vi "Begin.vi"(8 "error in":errorcluster) -> (0 "error out":errorcluster)   [LabVIEW 2019]
doc: "Called before other user functions, this VI is expected to open initial I/O refnums, load in file data, and do all program initialization. Notice that the <B>error out</B> terminal is simply used for data flow. Wiring it to other structures or subVIs ensures that this VI runs first."
uses:
  <vilib>/Rock Robotics/WPI/DriverStation/WPI_DriverStationRobotMode2.ctl
  <vilib>/Rock Robotics/WPI/Joystick/WPI_JoystickDeviceEnum.ctl
  <vilib>/Rock Robotics/SystemInterfaces/i2clib/i2c_bus.ctl
  <vilib>/Rock Robotics/WPI/Solenoid/WPI_SolenoidChannel.ctl
  <vilib>/Rock Robotics/WPI/ThirdParty/Phoenix-LabVIEW/Motor Controller/Controls/CTRE_Phoenix_MotorControl_LimitSwitchSource_Local.ctl
  <vilib>/Rock Robotics/WPI/ThirdParty/Phoenix-LabVIEW/Motor Controller/Controls/CTRE_Phoenix_MotorControl_LimitSwitchNormal.ctl
  <vilib>/Rock Robotics/SystemInterfaces/DIO/FPGA_DIOChannel.ctl
  Robot Global Data.vi
  <vilib>/Rock Robotics/Network Tables/NT Write String Array.vi
  <vilib>/Rock Robotics/WPI/Ultrasonic/WPI_SonarSRF04DigitalOpen.vi
  <vilib>/Rock Robotics/WPI/Ultrasonic/WPI_SonarSRF04DigitalRefNum Registry Set.vi
  <vilib>/Rock Robotics/WPI/Utilities/WPI_GetSetVariantRefNum.vi
  <vilib>/Rock Robotics/WPI/Switch/WPI_SwitchOpenLimit.vi
  <vilib>/Rock Robotics/WPI/Solenoid/WPI_SolenoidOpenDouble.vi
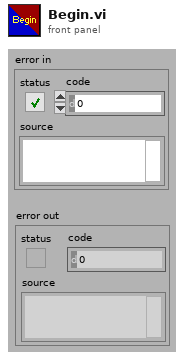
[diagram p1: front panel]
types:
  T1 = typedef "FPGA_DIOChannel.ctl" = enum8{"DIO 0", "DIO 1", "DIO 2", "DIO 3", "DIO 4", "DIO 5", "DIO 6", "DIO 7", "DIO 8", "DIO 9", "DIO MXP 0", "DIO MXP 1", "DIO MXP 2", "DIO MXP 3", "DIO MXP 4", "DIO MXP 5", "DIO MXP 6", "DIO MXP 7", "DIO MXP 8", "DIO MXP 9", "DIO MXP 10", "DIO MXP 11", "DIO MXP 12", "DIO MXP 13", "DIO MXP 14", "DIO MXP 15", "SPI Port CS1", "SPI Port CS2", "SPI Port CS3", "SPI Port MISO", "SPI Port MOSI", "Invalid"}
  T2 = typedef "WPI_SolenoidChannel.ctl" = enum8{"Solenoid 0", "Solenoid 1", "Solenoid 2", "Solenoid 3", "Solenoid 4", "Solenoid 5", "Solenoid 6", "Solenoid 7", "Invalid"}
  T3 = typedef "CTRE_Phoenix_MotorControl_LimitSwitchNormal.ctl" = enum16{"Normally Open", "Normally Closed", "Disabled"}
  T4 = typedef "CTRE_Phoenix_MotorControl_LimitSwitchSource_Local.ctl" = enum16{"Feedback Connector", "Remote Talon SRX", "Remote CANifier", "Deactivated"}
  T5 = typedef "WPI_JoystickDeviceEnum.ctl" = enum16{"USB 0", "USB 1", "USB 2", "USB 3", "USB 4", "USB 5"}
  T6 = typedef "i2c_bus.ctl" = enum16{"I2C On-Board", "I2C MXP", "Invalid"}
  T7 = typedef "WPI_DriverStationRobotMode2.ctl" = enum16{"Autonomous Disabled", "Autonomous Enabled", "Teleop Disabled", "Teleop Enabled", "Disconnected", "Finish", "Test Disabled", "Test Enabled", "Emergency Stopped"}
  T8 = typedef "WPI_CompressorDevRef.ctl" = cluster{"DevStatus":errorcluster, "Pneumatics Control Module":u8}
  T9 = typedef "WPI_SwitchDevRef.ctl" = cluster{"DevStatus":errorcluster, "DIO Channel":T1, "CntIndex":T10, "Normally Closed":bool}
  T10 = typedef "FPGA_CounterCtrSystemIndex.ctl" = enum8{"Ctr 0", "Ctr 1", "Ctr 2", "Ctr 3", "Ctr 4", "Ctr 5", "Ctr 6", "Ctr 7", "Invalid"}
  T11 = typedef "WPI_UltrasonicDeviceRef.ctl" = cluster{"DevStatus":errorcluster, "Ping Channel":T1, "Echo Channel":T1, "CntIndex":T10}
  T12 = typedef "Color Sensor V3 DevRef.ctl" = cluster{"I2CDevRef":T13}
  T13 = typedef "WPI_I2CDevRef.ctl" = cluster{"DevStatus":errorcluster, "Device Address":u8, "Handle":i32, "I2C Bus":T6}
  T14 = typedef "WPI_SolenoidDevRef.ctl" = cluster{"DevStatus":errorcluster, "Pneumatics Control Module":u8, "Forward Solenoid Channel":T2, "Reverse Solenoid Channel":T2}
  T15 = typedef "WPI_MotorControlDeviceRef.ctl" = cluster{"DeviceStatus":errorcluster, "Type":T16, "PWM":cluster{"PWM Channel":T17, "DeadBand":T18}, "CAN":cluster{"Device Number":u8, "SetOutput VI Ref":variant, "GetOutput VI Ref":variant, "Enable VI Ref":variant, "Disable VI Ref":variant, "Data":variant}, "Invert":bool, "DIO PWM":cluster{"PWM \"Enable\" Channel":T17, "DIOChannel":T1, "PWM Rate":dbl}}
  T16 = typedef "WPI_MotorControlType.ctl" = enum16{"PWM", "CAN", "DIO PWM"}
  T17 = typedef "FPGA_DIOPWMChannel.ctl" = enum8{"PWM 0", "PWM 1", "PWM 2", "PWM 3", "PWM 4", "PWM 5", "PWM 6", "PWM 7", "PWM 8", "PWM 9", "PWM MXP 0", "PWM MXP 1", "PWM MXP 2", "PWM MXP 3", "PWM MXP 4", "PWM MXP 5", "PWM MXP 6", "PWM MXP 7", "PWM MXP 8", "PWM MXP 9", "Invalid"}
  T18 = typedef "WPI_PWMDeadband.ctl" = cluster{"Name":string, "maxPositivePwm":i32, "minPositivePwm":i32, "centerPwm":i32, "maxNegativePwm":i32, "minNegativePwm":i32, "angularRange":u16}
  T19 = typedef "WPI_JoystickDevRef.ctl" = cluster{"Device":T5}
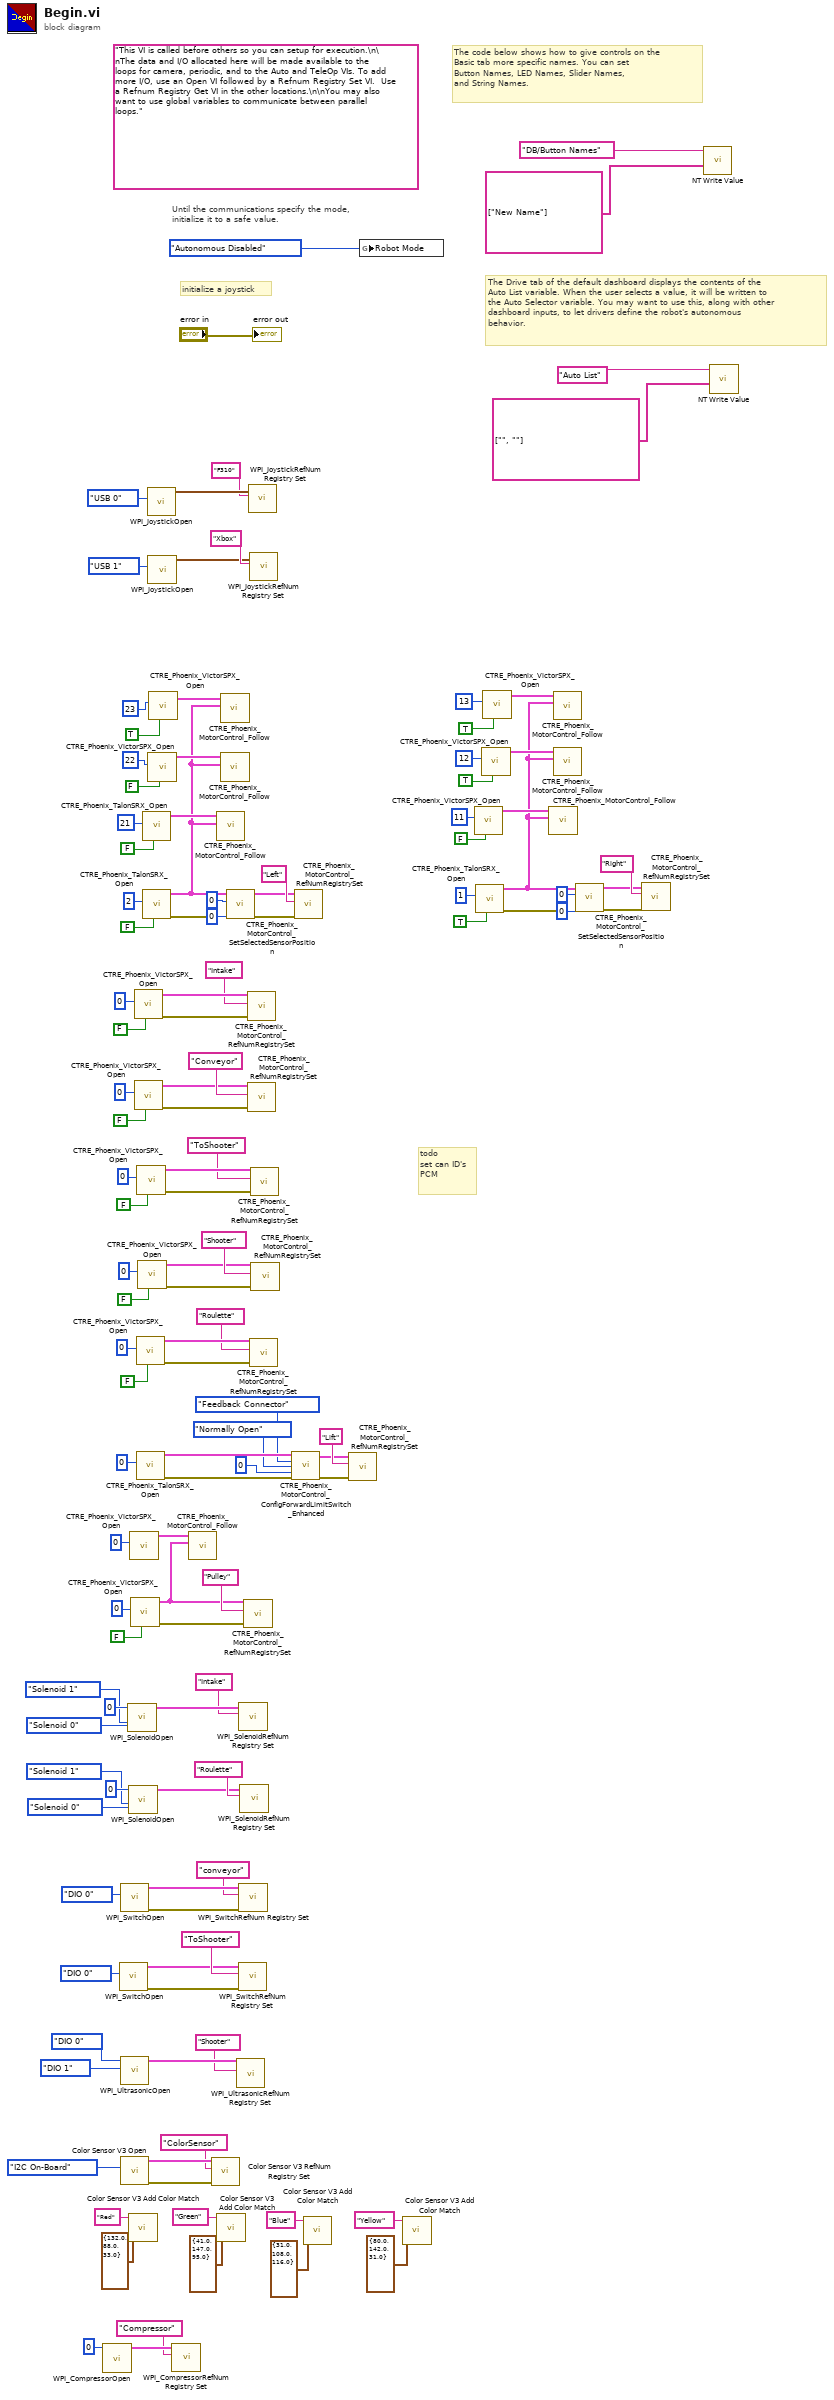
[diagram p0: block diagram]
diagram:
  (unwired) "This VI is called before others so you can setup for execution.\n\nThe data and I/O allocated here will be made available to the loops for camera, periodic, and to the Auto and TeleOp VIs. To add more I/O, use an Open VI followed by a Refnum Registry Set VI.  Use a Refnum Registry Get VI in the other locations.\n\nYou may also want to use global variables to communicate between parallel loops."
  # "todo\nset can ID's\nPCM"
  # "The Drive tab of the default dashboard displays the contents of the\nAuto List variable. When the user selects a value, it will be written to\nthe Auto Selector variable. You may want to use this, along with other\ndashboard inputs, to let drivers define the robot's autonomous\nbehavior."
  # "The code below shows how to give controls on the\nBasic tab more specific names. You can set\nButton Names, LED Names, Slider Names,\nand String Names."
  # "initialize a joystick"
  # "Until the communications specify the mode,\ninitialize it to a safe value."
  n1 = call <vilib>:"WPI_CompressorOpen.vi"("Pneumatics Control Module (0)"=u8 0) -> ("CompressorDevRef"=w11:T8)  [unwired: 13 in, 1 out]
  n2 = call-poly <vilib>:"WPI_SwitchOpen.vi"("DIO Channel"=FPGA_DIOChannel."DIO 0") -> ("error out"=w1:errorcluster, "SwitchDevRef"=w2:T9)  [unwired: 9 in]
  n3 = call-poly <vilib>:"WPI_SwitchOpen.vi"("DIO Channel"=FPGA_DIOChannel."DIO 0") -> ("error out"=w27:errorcluster, "SwitchDevRef"=w26:T9)  [unwired: 9 in]
  n4 = call-poly <vilib>:"WPI_UltrasonicOpen.vi"("Echo DIO Channel"=FPGA_DIOChannel."DIO 1", "Ping DIO Channel"=FPGA_DIOChannel."DIO 0") -> ("SonarSRF04DevRef"=w14:T11)  [unwired: 8 in, 1 out]
  n5 = call <vilib>:"Color Sensor V3 Open.vi"("I2C Bus"=i2c_bus."I2C On-Board") -> ("error out"=w84:errorcluster, "ColorSensorDevRef"=w83:T12)  [unwired: 9 in]
  n6 = call-poly <vilib>:"WPI_SolenoidOpen.vi"("Reverse Solenoid Channel"=WPI_SolenoidChannel."Solenoid 1", "Forward Solenoid Channel"=WPI_SolenoidChannel."Solenoid 0", "Pneumatics Control Module (0)"=u8 0) -> ("SolenoidDevRef"=w39:T14)  [unwired: 7 in, 1 out]
  n7 = call-poly <vilib>:"WPI_SolenoidOpen.vi"("Reverse Solenoid Channel"=WPI_SolenoidChannel."Solenoid 1", "Forward Solenoid Channel"=WPI_SolenoidChannel."Solenoid 0", "Pneumatics Control Module (0)"=u8 0) -> ("SolenoidDevRef"=w36:T14)  [unwired: 7 in, 1 out]
  n8 = call <vilib>:"Color Sensor V3 Add Color Match.vi"("Color"=cluster{"R":dbl, "G":dbl, "B":dbl} {"R"=132.0, "G"=88.0, "B"=33.0}, "Name"="Red") -> ()  [unwired: 10 in]
  n9 = call <vilib>:"CTRE_Phoenix_VictorSPX_Open.vi"("Device Number"=u8 0) -> ("CAN Talon SRX Ref"=w43:T15)  [unwired: 9 in, 1 out]
  n10 = call <vilib>:"CTRE_Phoenix_VictorSPX_Open.vi"("Invert"=FALSE, "Device Number"=u8 0) -> ("error out"=w45:errorcluster, "CAN Talon SRX Ref"=w42:T15)  [unwired: 8 in]
  n11 = call <vilib>:"CTRE_Phoenix_VictorSPX_Open.vi"("Invert"=FALSE, "Device Number"=u8 0) -> ("error out"=w92:errorcluster, "CAN Talon SRX Ref"=w91:T15)  [unwired: 8 in]
  n12 = call <vilib>:"CTRE_Phoenix_VictorSPX_Open.vi"("Invert"=FALSE, "Device Number"=u8 0) -> ("error out"=w60:errorcluster, "CAN Talon SRX Ref"=w61:T15)  [unwired: 8 in]
  n13 = call <vilib>:"CTRE_Phoenix_VictorSPX_Open.vi"("Invert"=FALSE, "Device Number"=u8 0) -> ("error out"=w30:errorcluster, "CAN Talon SRX Ref"=w29:T15)  [unwired: 8 in]
  n14 = call <vilib>:"CTRE_Phoenix_TalonSRX_Open.vi"("Device Number"=u8 0) -> ("error out"=w22:errorcluster, "CAN Talon SRX Ref"=w19:T15)  [unwired: 9 in]
  n15 = call <vilib>:"CTRE_Phoenix_VictorSPX_Open.vi"("Invert"=FALSE, "Device Number"=u8 0) -> ("error out"=w55:errorcluster, "CAN Talon SRX Ref"=w54:T15)  [unwired: 8 in]
  n16 = call <vilib>:"CTRE_Phoenix_VictorSPX_Open.vi"("Invert"=FALSE, "Device Number"=u8 0) -> ("error out"=w50:errorcluster, "CAN Talon SRX Ref"=w51:T15)  [unwired: 8 in]
  n17 = call <vilib>:"CTRE_Phoenix_TalonSRX_Open.vi"("Invert"=FALSE, "Device Number"=u8 21) -> ("CAN Talon SRX Ref"=w117:T15)  [unwired: 8 in, 1 out]
  n18 = call <vilib>:"CTRE_Phoenix_TalonSRX_Open.vi"("Invert"=FALSE, "Device Number"=u8 2) -> ("error out"=w65:errorcluster, "CAN Talon SRX Ref"=w68:T15)  [unwired: 8 in]
  n19 = call <vilib>:"WPI_JoystickOpen.vi"("JoystickDevice"=WPI_JoystickDeviceEnum."USB 0") -> ("JoystickDevRef"=w96:T19)  [unwired: 10 in]
  n20 = call <vilib>:"WPI_JoystickOpen.vi"("JoystickDevice"=WPI_JoystickDeviceEnum."USB 1") -> ("JoystickDevRef"=w72:T19)  [unwired: 10 in]
  n21 = call <vilib>:"CTRE_Phoenix_VictorSPX_Open.vi"("Invert"=FALSE, "Device Number"=u8 22) -> ("CAN Talon SRX Ref"=w112:T15)  [unwired: 8 in, 1 out]
  n22 = call <vilib>:"CTRE_Phoenix_VictorSPX_Open.vi"("Invert"=TRUE, "Device Number"=u8 23) -> ("CAN Talon SRX Ref"=w111:T15)  [unwired: 8 in, 1 out]
  n23 = call <vilib>:"WPI_CompressorRefNum Registry Set.vi"("refnum name"="Compressor", "CompressorDevRef"=w11) -> ()  [unwired: 8 in, 2 out]
  n24 = call <vilib>:"CTRE_Phoenix_MotorControl_Follow.vi"("Master Controller to Follow"=w42, "PhoenixMotorControlDevRef"=w43) -> ()  [unwired: 8 in, 2 out]
  n25 = call <vilib>:"Color Sensor V3 RefNum Registry Set.vi"("error in (no error)"=w84, "refnum name"="ColorSensor", "ColorSensorDevRef"=w83) -> ()  [unwired: 7 in, 2 out]
  n26 = call <vilib>:"CTRE_Phoenix_MotorControl_Follow.vi"("Master Controller to Follow"=w68, "PhoenixMotorControlDevRef"=w117) -> ()  [unwired: 8 in, 2 out]
  n27 = call <vilib>:"Color Sensor V3 Add Color Match.vi"("Color"=cluster{"R":dbl, "G":dbl, "B":dbl} {"R"=41.0, "G"=147.0, "B"=95.0}, "Name"="Green") -> ()  [unwired: 10 in]
  n28 = call <vilib>:"CTRE_Phoenix_MotorControl_Follow.vi"("Master Controller to Follow"=w68, "PhoenixMotorControlDevRef"=w111) -> ()  [unwired: 8 in, 2 out]
  n29 = call <vilib>:"CTRE_Phoenix_MotorControl_Follow.vi"("Master Controller to Follow"=w68, "PhoenixMotorControlDevRef"=w112) -> ()  [unwired: 8 in, 2 out]
  n30 = call <vilib>:"CTRE_Phoenix_MotorControl_SetSelectedSensorPosition.vi"("error in (no error)"=w65, "pidLoopIdx"=u32 0, "New Sensor Position"=0, "PhoenixMotorControlDevRef"=w68) -> ("error out"=w66:errorcluster, "PhoenixMotorControlDevRef"=w67:T15)  [unwired: 6 in]
  n31 = call-poly <vilib>:"WPI_UltrasonicRefNum Registry Set.vi"("refnum name"="Shooter", "SonarSRF04DevRef"=w14) -> ()  [unwired: 8 in, 2 out]
  n32 = call <vilib>:"WPI_SwitchRefNum Registry Set.vi"("error in (no error)"=w1, "refnum name"="ToShooter", "SwitchDevRef"=w2) -> ()  [unwired: 7 in, 2 out]
  n33 = call <vilib>:"WPI_SolenoidRefNum Registry Set.vi"("refnum name"="Intake", "SolenoidDevRef"=w39) -> ()  [unwired: 8 in, 2 out]
  n34 = call <vilib>:"WPI_SwitchRefNum Registry Set.vi"("error in (no error)"=w27, "refnum name"="conveyor", "SwitchDevRef"=w26) -> ()  [unwired: 7 in, 2 out]
  n35 = call <vilib>:"WPI_SolenoidRefNum Registry Set.vi"("refnum name"="Roulette", "SolenoidDevRef"=w36) -> ()  [unwired: 8 in, 2 out]
  n36 = call <vilib>:"CTRE_Phoenix_MotorControl_RefNumRegistrySet.vi"("error in (no error)"=w45, "refnum name"="Pulley", "PhoenixMotorControlDevRef"=w42) -> ()  [unwired: 7 in, 2 out]
  n37 = call <vilib>:"CTRE_Phoenix_MotorControl_RefNumRegistrySet.vi"("error in (no error)"=w92, "refnum name"="Intake", "PhoenixMotorControlDevRef"=w91) -> ()  [unwired: 7 in, 2 out]
  n38 = call <vilib>:"CTRE_Phoenix_MotorControl_RefNumRegistrySet.vi"("error in (no error)"=w60, "refnum name"="Conveyor", "PhoenixMotorControlDevRef"=w61) -> ()  [unwired: 7 in, 2 out]
  n39 = call <vilib>:"WPI_JoystickRefNum Registry Set.vi"("refnum name"="F310", "JoystickDevRef"=w96) -> ()  [unwired: 8 in, 2 out]
  n40 = call <vilib>:"WPI_JoystickRefNum Registry Set.vi"("refnum name"="Xbox", "JoystickDevRef"=w72) -> ()  [unwired: 8 in, 2 out]
  n41 = call <vilib>:"CTRE_Phoenix_MotorControl_RefNumRegistrySet.vi"("error in (no error)"=w30, "refnum name"="Roulette", "PhoenixMotorControlDevRef"=w29) -> ()  [unwired: 7 in, 2 out]
  n42 = call <vilib>:"CTRE_Phoenix_MotorControl_RefNumRegistrySet.vi"("error in (no error)"=w55, "refnum name"="ToShooter", "PhoenixMotorControlDevRef"=w54) -> ()  [unwired: 7 in, 2 out]
  n43 = call <vilib>:"CTRE_Phoenix_MotorControl_RefNumRegistrySet.vi"("error in (no error)"=w50, "refnum name"="Shooter", "PhoenixMotorControlDevRef"=w51) -> ()  [unwired: 7 in, 2 out]
  n44 = call <vilib>:"CTRE_Phoenix_MotorControl_ConfigForwardLimitSwitch_Enhanced.vi"("PhoenixMotorControlDevRef"=w19, "Limit Switch Source"=CTRE_Phoenix_MotorControl_LimitSwitchSource_Local."Feedback Connector", "NormallyOpenOrClosed"=CTRE_Phoenix_MotorControl_LimitSwitchNormal."Normally Open", "deviceID"=0, "error in (no error)"=w22) -> ("PhoenixMotorControlDevRef"=w20:T15, "error out"=w21:errorcluster)  [unwired: 9 in]
  n45 = call <vilib>:"CTRE_Phoenix_MotorControl_RefNumRegistrySet.vi"("error in (no error)"=w66, "refnum name"="Left", "PhoenixMotorControlDevRef"=w67) -> ()  [unwired: 7 in, 2 out]
  n46 = call <vilib>:"Color Sensor V3 Add Color Match.vi"("Color"=cluster{"R":dbl, "G":dbl, "B":dbl} {"R"=31.0, "G"=108.0, "B"=116.0}, "Name"="Blue") -> ()  [unwired: 10 in]
  n47 = call <vilib>:"CTRE_Phoenix_MotorControl_RefNumRegistrySet.vi"("error in (no error)"=w21, "refnum name"="Lift", "PhoenixMotorControlDevRef"=w20) -> ()  [unwired: 7 in, 2 out]
  n48 = global write "Robot Global Data.vi" "Robot Mode"(WPI_DriverStationRobotMode2."Autonomous Disabled" ("Robot Mode")) -> ()
  n49 = call <vilib>:"Color Sensor V3 Add Color Match.vi"("Color"=cluster{"R":dbl, "G":dbl, "B":dbl} {"R"=80.0, "G"=142.0, "B"=31.0}, "Name"="Yellow") -> ()  [unwired: 10 in]
  n50 = call <vilib>:"CTRE_Phoenix_VictorSPX_Open.vi"("Invert"=FALSE, "Device Number"=u8 11) -> ("CAN Talon SRX Ref"=w100:T15)  [unwired: 8 in, 1 out]
  n51 = call <vilib>:"CTRE_Phoenix_TalonSRX_Open.vi"("Invert"=TRUE, "Device Number"=u8 1) -> ("error out"=w64:errorcluster, "CAN Talon SRX Ref"=w89:T15)  [unwired: 8 in]
  n52 = call <vilib>:"CTRE_Phoenix_VictorSPX_Open.vi"("Invert"=TRUE, "Device Number"=u8 12) -> ("CAN Talon SRX Ref"=w109:T15)  [unwired: 8 in, 1 out]
  n53 = call <vilib>:"CTRE_Phoenix_VictorSPX_Open.vi"("Invert"=TRUE, "Device Number"=u8 13) -> ("CAN Talon SRX Ref"=w110:T15)  [unwired: 8 in, 1 out]
  n54 = call <vilib>:"CTRE_Phoenix_MotorControl_Follow.vi"("Master Controller to Follow"=w89, "PhoenixMotorControlDevRef"=w100) -> ()  [unwired: 8 in, 2 out]
  n55 = call <vilib>:"CTRE_Phoenix_MotorControl_Follow.vi"("Master Controller to Follow"=w89, "PhoenixMotorControlDevRef"=w110) -> ()  [unwired: 8 in, 2 out]
  n56 = call <vilib>:"CTRE_Phoenix_MotorControl_Follow.vi"("Master Controller to Follow"=w89, "PhoenixMotorControlDevRef"=w109) -> ()  [unwired: 8 in, 2 out]
  n57 = call <vilib>:"CTRE_Phoenix_MotorControl_SetSelectedSensorPosition.vi"("error in (no error)"=w64, "pidLoopIdx"=u32 0, "New Sensor Position"=0, "PhoenixMotorControlDevRef"=w89) -> ("error out"=w63:errorcluster, "PhoenixMotorControlDevRef"=w88:T15)  [unwired: 6 in]
  n58 = call <vilib>:"CTRE_Phoenix_MotorControl_RefNumRegistrySet.vi"("error in (no error)"=w63, "refnum name"="Right", "PhoenixMotorControlDevRef"=w88) -> ()  [unwired: 7 in, 2 out]
  n59 = call-poly <vilib>:"NT Write Value.vi"("String Array"=string[] ["New Name"], "Name"="DB/Button Names") -> ()  [unwired: 9 in, 1 out]
  n60 = call-poly <vilib>:"NT Write Value.vi"("String Array"=string[] ["", ""], "Name"="Auto List") -> ()  [unwired: 9 in, 1 out]
  "error out" <- "error in"
